vi "VI_Open.vi"(8 "Panel Bounds":T1={"Left"=200, "Top"=200, "Right"=500, "Bottom"=500}, 9 "Строка help":string="Тестовая строка", 11 "Current VI In":refnum<vi>) -> (3 "Current VI Out":refnum<vi>)   [LabVIEW 2015]
uses:
  <vilib>/Utility/miscctls.llb/LVRectTypeDef.ctl
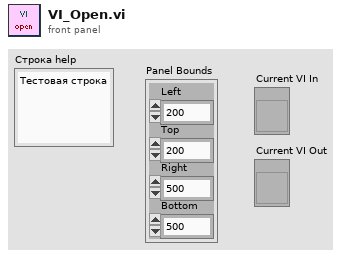
[diagram p1: front panel]
types:
  T1 = typedef "LVRectTypeDef.ctl" = cluster{"Left":i16, "Top":i16, "Right":i16, "Bottom":i16}
  T2 = enum32{"Bad", "Idle", "Run top level", "Running"}
  T3 = enum32{"Invalid", "Standard", "Closed", "Hidden", "Minimized", "Maximized"}
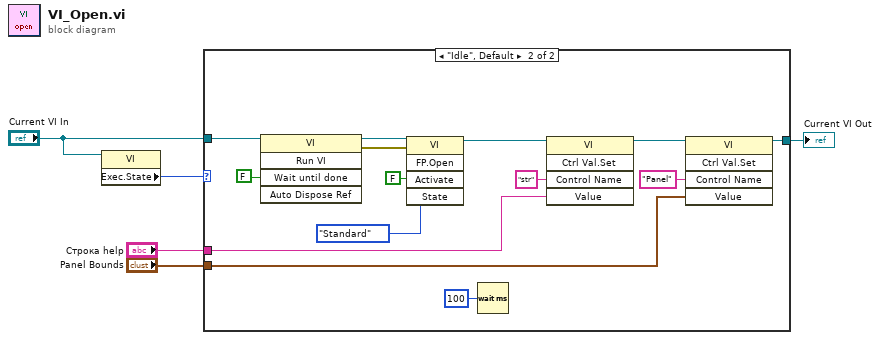
[diagram p0: block diagram]
diagram:
  n1 = property class="VI"(reference="Current VI In") -> ("Exec.State"=w1:T2)  [unwired: 1 in, 2 out]
  n2 = case shown="\"Idle\", Default" w1 {
    tunnel: "Строка help" -> [_ w13]
    tunnel: "Panel Bounds" -> [_ w10]
    tunnel: [w6 w9] -> w3
    tunnel: "Current VI In" -> [w6 w8]
    frame "Run top level", "Running" {
    }
    frame "Idle", Default {
      n3 = invoke class="VI" method="Run VI"(reference=w8, "Wait until done"=FALSE) -> (reference out=w20:refnum<vi>, error out=w19:errorcluster)  [unwired: 3 in, 3 out]
      n4 = invoke class="VI" method="FP.Open"(reference=w20, error in=w19, "Activate"=FALSE, "State"=T3."Standard") -> (reference out=w15:refnum<vi>)  [unwired: 1 in, 4 out]
      n5 = Wait (ms)(milliseconds to wait=u32 100) -> ()  [unwired: 1 out]
      n6 = invoke class="VI" method="Ctrl Val.Set"(reference=w15, "Control Name"="str", "Value"=w13) -> (reference out=w12:refnum<vi>)  [unwired: 2 in, 4 out]
      n7 = invoke class="VI" method="Ctrl Val.Set"(reference=w12, "Control Name"="Panel", "Value"=w10) -> (reference out=w9:refnum<vi>)  [unwired: 2 in, 4 out]
    }
  }
  "Current VI Out" <- w3
